vi "Update Order Number.vi"(8 "error in (no error)":errorcluster, 10 "Order Number":u32, 11 "Customer In":refnum<class "Customer.lvclass">) -> (0 "error out":errorcluster, 3 "Customer Out":refnum<class "Customer.lvclass">)   [LabVIEW 2020, in "Customer.lvclass"]
uses:
  Customer.lvclass
  C:/Program Files (x86)/National Instruments/LabVIEW 2020/vi.lib/Asteme/Triarc Framework/Process/Process.lvclass
  <vilib>/Asteme/Triarc Framework/Process/Process.lvclass/Process.ctl
  <vilib>/AdvancedString/1D String Array to Delimited String.vi
  <vilib>/Asteme/Triarc Framework/Process/Public/Lifecycle/Get Lifecycle State.vi
  <vilib>/Utility/error.llb/Clear Errors.vi
  <vilib>/Utility/error.llb/Error Cluster From Error Code.vi
  <vilib>/Asteme/Triarc Framework/Process/Process.lvclass
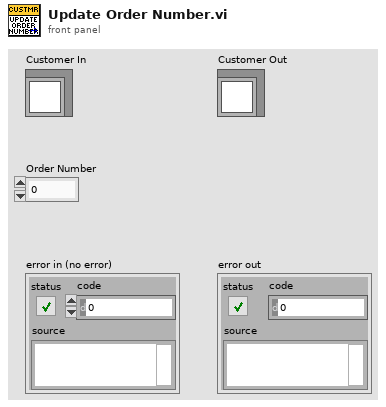
[diagram p1: front panel]
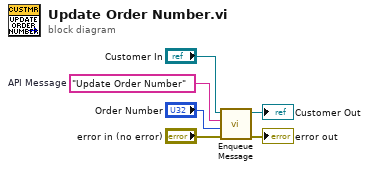
[diagram p0: block diagram]
diagram:
  w3 = "Update Order Number"  # API Message
  n1 = call <vilib>:"Enqueue Message.vi"("error in (no error)"="error in (no error)", "Message Data"="Order Number", "Message"=w3, "Process In"="Customer In") -> ("error out"=→"error out":errorcluster, "Process Out"=→"Customer Out":refnum<class "Customer.lvclass">)  [unwired: 6 in]
